vi "CVT name.vi"() -> ()   [LabVIEW 2017, in "Toolbox.lvlib"]
uses:
  Toolbox.lvlib
panel:
  in  "Row4 Match":string="Row4 Match"
  in  "Row3 Match":string="Row3 Match"
  in  "Row2 Match":string="Row2 Match"
  in  "Find Center":string="Center Edge"
  in  "Row1 Match":string="Row1 Match"
  in  "Find Ering":string="Ering Edge"
  # "Judgement"
  # "Find Edge ROI"
  # "Match ROI"
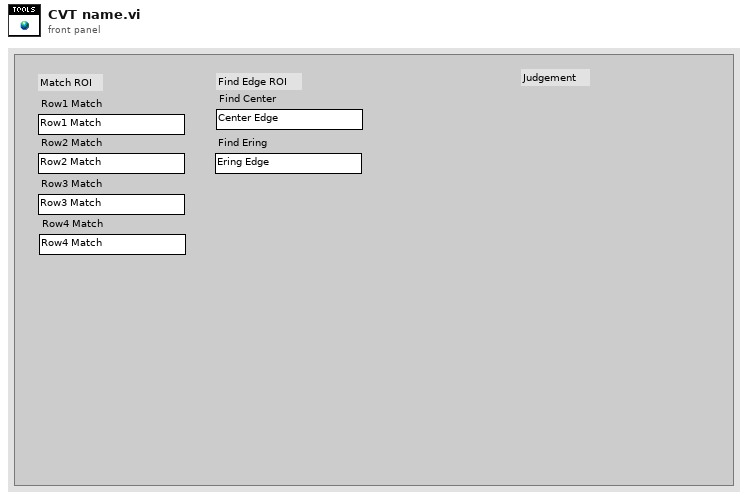
[diagram p1: front panel]
diagram:
